vi "Configure Display Basic.vi"(0 "VISA resource name":refnum<visa-resource-name>, 5 "Background Color (1: White)":u16(ring)=1 items=["Black", "White"], 7 "Scroll Time (1: 10s)":u16(ring)=1 items=["5s", "10s", "20s", "30s", "1min"], 9 "Jump Default Display (0: Off)":u16(ring) items=["Off", "1min", "2min", "5min", "10min", "20min", "30min", "1h"], 11 "error in (no error)":errorcluster) -> (4 "VISA resource name out":refnum<visa-resource-name>, 15 "error out":errorcluster)   [LabVIEW 2020, in "Yokogawa GX Series.lvlib"]
doc: "Sets the display background color, scroll time and auto jump.\n\nCommands: SBackColor, SGrpChange, SAutoJump\n\nNote: This VI does nothing when the instrument is GM10."
uses:
  <instrlib>/Yokogawa GX Series/Yokogawa GX Series.lvlib
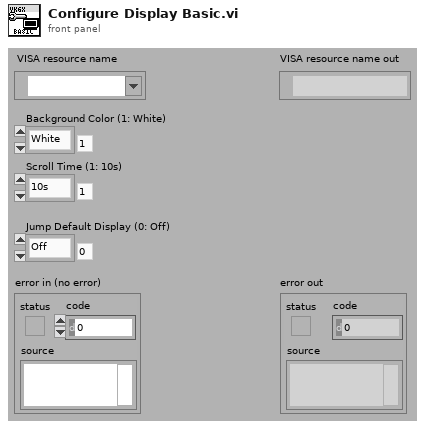
[diagram p1: front panel]
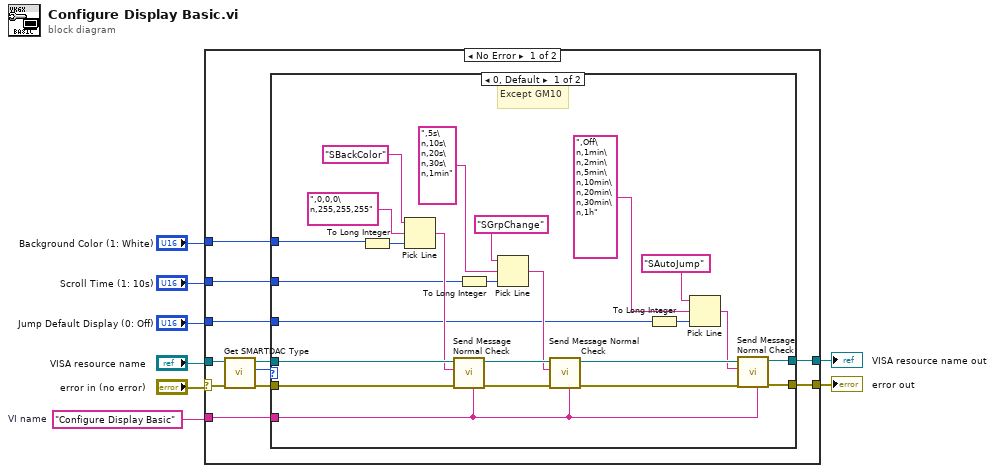
[diagram p0: block diagram]
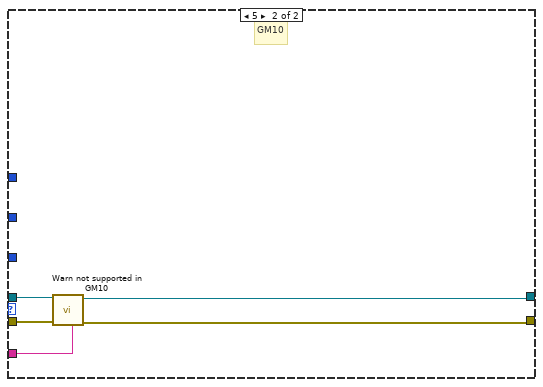
[diagram p2: hidden frame]
diagram:
  w3 = "Configure Display Basic"  # VI name
  n1 = case shown="No Error" "error in (no error)" {
    selector: "error in (no error)" -> [w12 w49]
    tunnel: "VISA resource name" -> [w13 w50]
    tunnel: "Scroll Time (1: 10s)" -> [w19 _]
    tunnel: "Jump Default Display (0: Off)" -> [w18 _]
    tunnel: [w17 w50] -> w5
    tunnel: [w16 w49] -> w4
    tunnel: w3 -> [w15 _]
    tunnel: "Background Color (1: White)" -> [w14 _]
    frame No Error {
      n2 = call <instrlib>:"Get SMARTDAC Type.vi"("error in (no error)"=w12, "VISA resource name"=w13) -> ("error out"=w10:errorcluster, "SMARTDAC+ Type"=w9:u16, "VISA resource name out"=w11:refnum<visa-resource-name>)  [unwired: 7 in]
      n3 = case shown="0, Default" w9 {
        tunnel: w11 -> [w43 w48]
        tunnel: w19 -> [w22 _]
        tunnel: w18 -> [w20 _]
        tunnel: [w32 w46] -> w17
        tunnel: [w31 w45] -> w16
        tunnel: w15 -> [w30 w44]
        tunnel: w14 -> [w24 _]
        tunnel: w10 -> [w27 w47]
        frame 0, Default {
          # "Except GM10"
          n4 = To Long Integer(number=w24) -> (32bit integer=w25:i32)
          n5 = Pick Line(string ("")="SBackColor", multi-line string=",0,0,0\n,255,255,255", line index=w25) -> (output string=w29:string)
          n6 = call <instrlib>:"Send Message Normal Check.vi"("Source (\"\")"=w30, "error in (no error)"=w27, "Send Message (\"\")"=w29, "VISA resource name"=w43) -> ("error out"=w39:errorcluster, "VISA resource name out"=w40:refnum<visa-resource-name>)  [unwired: 2 in, 4 out]
          n7 = To Long Integer(number=w22) -> (32bit integer=w23:i32)
          n8 = Pick Line(string ("")="SGrpChange", multi-line string=",5s\n,10s\n,20s\n,30s\n,1min", line index=w23) -> (output string=w38:string)
          n9 = call <instrlib>:"Send Message Normal Check.vi"("Source (\"\")"=w30, "error in (no error)"=w39, "Send Message (\"\")"=w38, "VISA resource name"=w40) -> ("error out"=w34:errorcluster, "VISA resource name out"=w35:refnum<visa-resource-name>)  [unwired: 2 in, 4 out]
          n10 = To Long Integer(number=w20) -> (32bit integer=w21:i32)
          n11 = Pick Line(string ("")="SAutoJump", multi-line string=",Off\n,1min\n,2min\n,5min\n,10min\n,20min\n,30min\n,1h", line index=w21) -> (output string=w33:string)
          n12 = call <instrlib>:"Send Message Normal Check.vi"("Source (\"\")"=w30, "error in (no error)"=w34, "Send Message (\"\")"=w33, "VISA resource name"=w35) -> ("error out"=w31:errorcluster, "VISA resource name out"=w32:refnum<visa-resource-name>)  [unwired: 2 in, 4 out]
        }
        frame 5 {
          # "GM10"
          n13 = call <instrlib>:"Warn not supported in GM10.vi"("Source (\"\")"=w44, "error in (no error)"=w47, "VISA resource name"=w48) -> ("error out"=w45:errorcluster, "VISA resource name out"=w46:refnum<visa-resource-name>)  [unwired: 7 in]
        }
      }
    }
    frame Error {
    }
  }
  "error out" <- w4
  "VISA resource name out" <- w5
